vi "Change Copy LLB to NI VeriStand.vi"(7 "CD Execution Mode":T1=enum."Inline Model Interface", 8 "error in (no error)":errorcluster, 10 "Copy .LLB to ... path":path, 11 "CD Name":string) -> (0 "error out":errorcluster)   [LabVIEW 2014, in "CD model script.lvlib"]
doc: "Change the block diagram of \"Copy .LLB to NI VeriStand dir\" accoding to the custom device name and the execution mode."
uses:
  CD model script.lvlib
  CD Wizard - Execution Mode.ctl
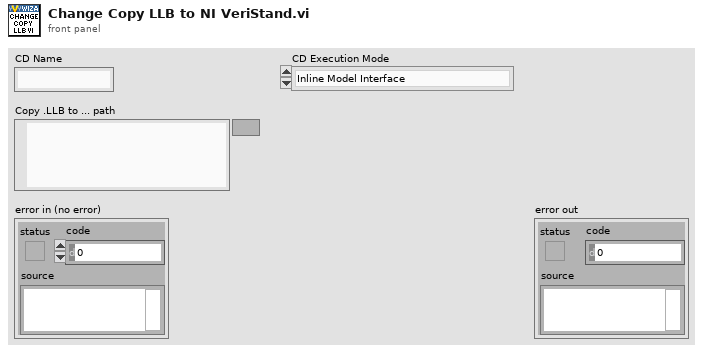
[diagram p1: front panel]
types:
  T1 = typedef "CD model script.lvlib/CD Wizard - Execution Mode.ctl" = enum16{"Asynchronous", "Inline HW Interface", "Inline Model Interface", "Inline Timing and Sync", "Asynchronous Timing and Sync"}
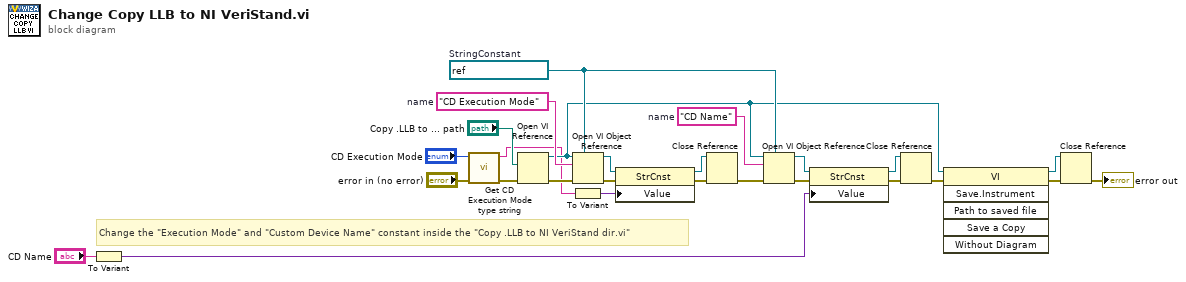
[diagram p0: block diagram]
diagram:
  w15 = "CD Name"  # name
  w23 = "CD Execution Mode"  # name
  w16 = refnum<vi> refnum  # StringConstant
  # "Change the \"Execution Mode\" and \"Custom Device Name\" constant inside the \"Copy .LLB to NI VeriStand dir.vi\""
  n1 = To Variant(anything="CD Name") -> (Variant=w10:variant)
  n2 = call "Get CD Execution Mode type string.vi"("error in (no error)"="error in (no error)", "CD Execution Mode"="CD Execution Mode") -> ("error out"=w4:errorcluster, "Execution Mode type"=w3:string)  [unwired: 8 in]
  n3 = Open VI Reference(vi path="Copy .LLB to ... path", error in (no error)=w4) -> (vi reference=w7:refnum<vi>, error out=w5:errorcluster)  [unwired: 4 in]
  n4 = Open VI Object Reference(7:w16, 8:w5, 10:w23, 11:w7) -> (0:w22:errorcluster, 3:w19:refnum<vi>)
  n5 = To Variant(anything=w3) -> (Variant=w18:variant)
  n6 = property class="StrCnst"(reference=w19, error in=w22, "Value"=w18) -> (reference out=w21:refnum<vi>, error out=w20:errorcluster)
  n7 = Close Reference(reference=w21, error in (no error)=w20) -> (error out=w17:errorcluster)
  n8 = Open VI Object Reference(7:w16, 8:w17, 10:w15, 11:w7) -> (0:w14:errorcluster, 3:w13:refnum<vi>)
  n9 = property class="StrCnst"(reference=w13, error in=w14, "Value"=w10) -> (reference out=w8:refnum<vi>, error out=w9:errorcluster)
  n10 = Close Reference(reference=w8, error in (no error)=w9) -> (error out=w6:errorcluster)
  n11 = invoke class="VI" method="Save.Instrument"(reference=w7, error in=w6) -> (reference out=w12:refnum<vi>, error out=w11:errorcluster)  [unwired: 4 in, 4 out]
  n12 = Close Reference(reference=w12, error in (no error)=w11) -> (error out=→"error out":errorcluster)
